vi "Lab05 JohnDoldol.vi"() -> ()   [LabVIEW 2016]
uses:
  <vilib>/DAQmx/read.llb/DAQmx Read (Analog DBL 1Chan 1Samp).vi
panel:
  out "Vo":dbl
  in  "stop 2":bool
  out "Thermometer":dbl(slide) scale=0.0..100.0
  out "Waveform Chart":dbl(graph)
  out "data":dbl format="%0.2f"
  in  "task/channels in":refnum<k21>
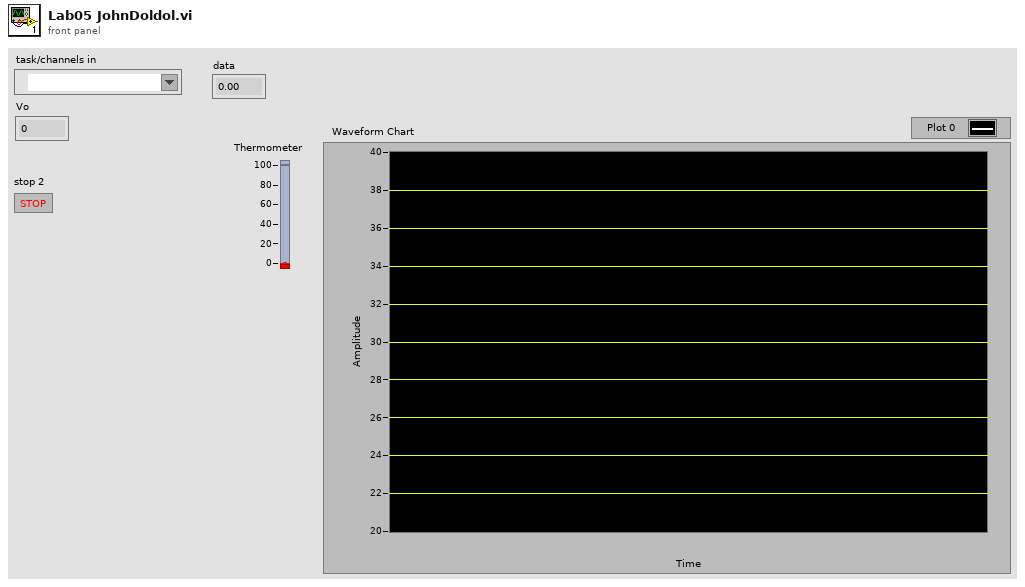
[diagram p1: front panel]
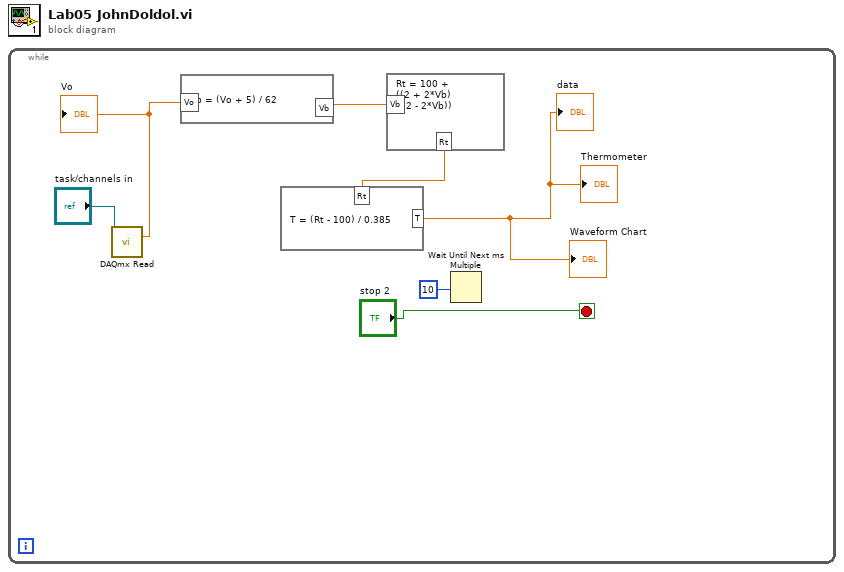
[diagram p0: block diagram]
diagram:
  n1 = while {
    stop <- "stop 2" stop-if-true
    n2 = call-poly <vilib>:"DAQmx Read.vi"("task/channels in"="task/channels in") -> ("data"=w1:dbl)  [unwired: 12 in, 2 out]
    "Vo" <- w1
    n3 = formula code="Vb = (Vo + 5) / 62"("Vo"=w1) -> ("Vb"=w3:dbl)
    n4 = formula code="Rt = 100 + \n((2 + 2*Vb) \n/ (2 - 2*Vb))"("Vb"=w3) -> ("Rt"=w2:dbl)
    n5 = formula code="T = (Rt - 100) / 0.385"("Rt"=w2) -> ("T"=→"data" →"Waveform Chart" →"Thermometer":dbl)
    n6 = Wait Until Next ms Multiple(millisecond multiple=10) -> ()  [unwired: 1 out]
  }
